vi "SetExpFeed.vi"   [LabVIEW 2012]
uses:
  <vilib>/Rock Robotics/WPI/Camera/WPI_CameraExposure Values.ctl
panel:
  # "This vi sets exposure for driver station camera feed"
types:
  T1 = typedef "WPI_CameraExposure Values.ctl" = enum16{"Auto", "Flicker-free 50 Hz", "Flicker-free 60 Hz", "Hold current"}
  T2 = typedef "WPI_CameraDevRef.ctl" = cluster{"Camera Address":string, "CameraStatus":errorcluster, "Acquire Image Notifier":refnum<notifier>}
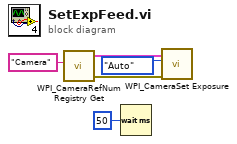
[diagram p0: block diagram]
diagram:
  n1 = call <vilib>:"WPI_CameraRefNum Registry Get.vi"("refnum name"="Camera") -> ("error out"=w3:errorcluster, "CameraDevRef"=w4:T2)  [unwired: 9 in]
  n2 = Wait (ms)(milliseconds to wait=u32 50) -> ()  [unwired: 1 out]
  n3 = call <vilib>:"WPI_CameraSet Exposure.vi"("error in (no error)"=w3, "Exposure"=WPI_CameraExposure_Values."Auto", "CameraDevRef"=w4) -> ()  [unwired: 7 in, 2 out]
